vi "Read Math.vi"(0 "VISA resource name":refnum<visa-resource-name>, 11 "error in (no error)":errorcluster) -> (2 "Maximum":dbl, 3 "Average":dbl, 4 "VISA resource name out":refnum<visa-resource-name>, 6 "Pass/Fail":bool, 8 "dB":dbl, 10 "dBm":dbl, 13 "Minimum":dbl, 14 "Count":u32, 15 "error out":errorcluster)   [LabVIEW 2020, in "Library Instrument & Equipement.lvlib" / "Library Multimeter.lvlib" / "RIGOL DM3058.lvlib"]
doc: "Read (Math) returns the Maximum, Minimum, Average, Count, dB, dBm and Pass/Fail value from multiple measurements."
uses:
  RIGOL DM3058.lvlib
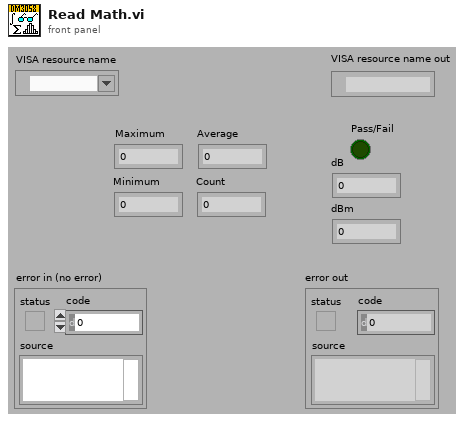
[diagram p1: front panel]
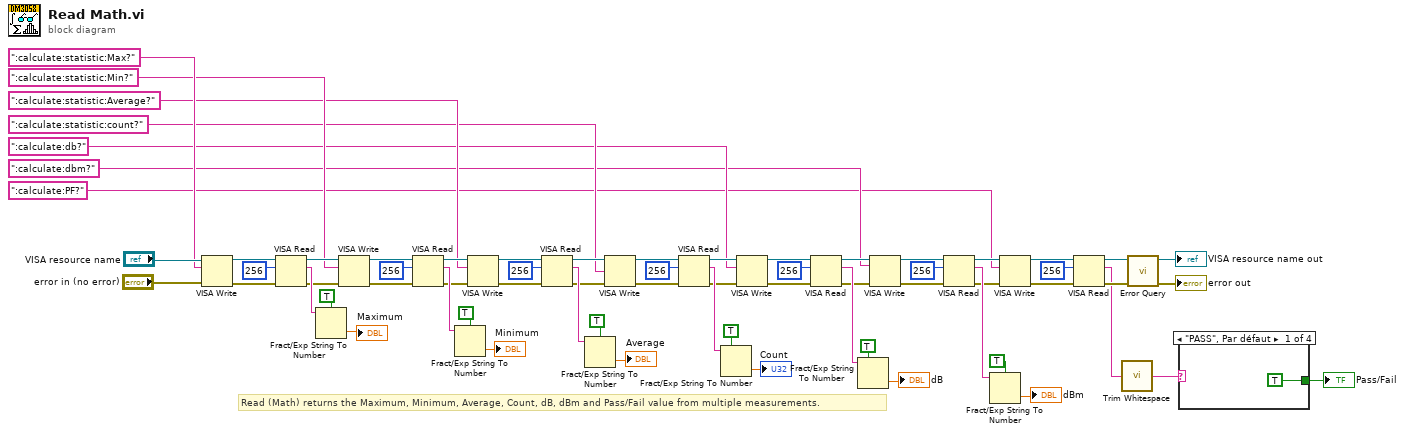
[diagram p0: block diagram]
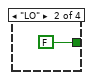
[diagram p2: hidden frame]
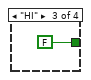
[diagram p3: hidden frame]
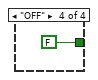
[diagram p4: hidden frame]
diagram:
  # "Read (Math) returns the Maximum, Minimum, Average, Count, dB, dBm and Pass/Fail value from multiple measurements."
  n1 = VISA Write(VISA resource name="VISA resource name", write buffer=":calculate:statistic:Max?", error in (no error)="error in (no error)") -> (VISA resource name out=w66:refnum<visa-resource-name>, error out=w65:errorcluster)  [unwired: 1 out]
  n2 = VISA Read(VISA resource name=w66, byte count=u32 256 ("字节总数"), error in (no error)=w65) -> (VISA resource name out=w56:refnum<visa-resource-name>, read buffer=w61:string, error out=w55:errorcluster)  [unwired: 1 out]
  n3 = Fract/Exp String To Number(use system decimal point (T)=TRUE, string=w61) -> (number=→"Maximum":dbl)  [unwired: 3 out]
  n4 = VISA Write(VISA resource name=w56, write buffer=":calculate:statistic:Min?", error in (no error)=w55) -> (VISA resource name out=w58:refnum<visa-resource-name>, error out=w59:errorcluster)  [unwired: 1 out]
  n5 = VISA Read(VISA resource name=w58, byte count=u32 256 ("字节总数"), error in (no error)=w59) -> (VISA resource name out=w48:refnum<visa-resource-name>, read buffer=w53:string, error out=w47:errorcluster)  [unwired: 1 out]
  n6 = Fract/Exp String To Number(use system decimal point (T)=TRUE, string=w53) -> (number=→"Minimum":dbl)  [unwired: 3 out]
  n7 = VISA Write(VISA resource name=w48, write buffer=":calculate:statistic:Average?", error in (no error)=w47) -> (VISA resource name out=w50:refnum<visa-resource-name>, error out=w49:errorcluster)  [unwired: 1 out]
  n8 = VISA Read(VISA resource name=w50, byte count=u32 256 ("字节总数"), error in (no error)=w49) -> (VISA resource name out=w38:refnum<visa-resource-name>, read buffer=w45:string, error out=w39:errorcluster)  [unwired: 1 out]
  n9 = Fract/Exp String To Number(use system decimal point (T)=TRUE, string=w45) -> (number=→"Average":dbl)  [unwired: 3 out]
  n10 = VISA Write(VISA resource name=w38, write buffer=":calculate:statistic:count?", error in (no error)=w39) -> (VISA resource name out=w41:refnum<visa-resource-name>, error out=w42:errorcluster)  [unwired: 1 out]
  n11 = VISA Read(VISA resource name=w41, byte count=u32 256 ("字节总数"), error in (no error)=w42) -> (VISA resource name out=w32:refnum<visa-resource-name>, read buffer=w36:string, error out=w31:errorcluster)  [unwired: 1 out]
  n12 = Fract/Exp String To Number(use system decimal point (T)=TRUE, string=w36) -> (number=→"Count":dbl)  [unwired: 3 out]
  n13 = VISA Write(VISA resource name=w32, write buffer=":calculate:db?", error in (no error)=w31) -> (VISA resource name out=w34:refnum<visa-resource-name>, error out=w33:errorcluster)  [unwired: 1 out]
  n14 = VISA Read(VISA resource name=w34, byte count=u32 256 ("字节总数"), error in (no error)=w33) -> (VISA resource name out=w24:refnum<visa-resource-name>, read buffer=w30:string, error out=w23:errorcluster)  [unwired: 1 out]
  n15 = Fract/Exp String To Number(use system decimal point (T)=TRUE, string=w30) -> (number=→"dB":dbl)  [unwired: 3 out]
  n16 = VISA Write(VISA resource name=w24, write buffer=":calculate:dbm?", error in (no error)=w23) -> (VISA resource name out=w26:refnum<visa-resource-name>, error out=w27:errorcluster)  [unwired: 1 out]
  n17 = VISA Read(VISA resource name=w26, byte count=u32 256 ("字节总数"), error in (no error)=w27) -> (VISA resource name out=w15:refnum<visa-resource-name>, read buffer=w20:string, error out=w16:errorcluster)  [unwired: 1 out]
  n18 = Fract/Exp String To Number(use system decimal point (T)=TRUE, string=w20) -> (number=→"dBm":dbl)  [unwired: 3 out]
  n19 = VISA Write(VISA resource name=w15, write buffer=":calculate:PF?", error in (no error)=w16) -> (VISA resource name out=w18:refnum<visa-resource-name>, error out=w17:errorcluster)  [unwired: 1 out]
  n20 = VISA Read(VISA resource name=w18, byte count=u32 256 ("字节总数"), error in (no error)=w17) -> (VISA resource name out=w12:refnum<visa-resource-name>, read buffer=w1:string, error out=w11:errorcluster)  [unwired: 1 out]
  n21 = call <vilib>:"Trim Whitespace.vi"("string"=w1) -> ("trimmed string"=w2:string)  [unwired: 1 in]
  n22 = call "Error Query.vi"("error in (no error)"=w11, "VISA resource name"=w12) -> ("error out"=→"error out":errorcluster, "VISA resource name out"=→"VISA resource name out":refnum<visa-resource-name>)  [unwired: 6 in, 2 out]
  n23 = case shown="\"PASS\", Par défaut" w2 {
    tunnel: [TRUE FALSE FALSE FALSE] -> w13
    frame "PASS", Default {
    }
    frame "LO" {
    }
    frame "HI" {
    }
    frame "OFF" {
    }
  }
  "Pass/Fail" <- w13
